vi "9608 Invalid PDO Communication Parameter Type--error.vi"(8 "error in (no error)":errorcluster, 11 "Type":enum16{"TPDO", "RPDO"}(ring)) -> (0 "error out":errorcluster)   [LabVIEW 2024, in "Electronic Datasheet.lvlib"]
uses:
  Electronic Datasheet.lvlib
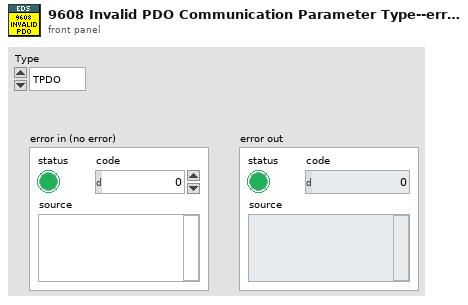
[diagram p1: front panel]
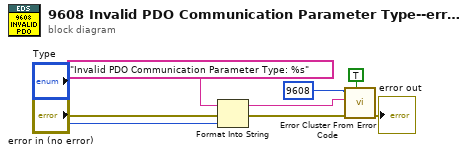
[diagram p0: block diagram]
diagram:
  n1 = Format Into String(initial string="Invalid PDO Communication Parameter Type: %s" ("error message (\"\")"), error in="error in (no error)", "Type") -> (resulting string=w6:string, error out=w4:errorcluster)  [unwired: 1 in]
  n2 = call <vilib>:"Error Cluster From Error Code.vi"("show call chain? (False)"=TRUE, "error in (no error)"=w4, "error message (\"\")"=w6, "error code (0)"=9608) -> ("error out"=→"error out":errorcluster)  [unwired: 5 in]
